vi "makeDecisions.vi"(8 "error in (no error)":errorcluster, 10 "model":refnum<class "Model.lvclass">, 11 "WaitingForSettledPState in":refnum<class "WaitingForSettledPState.lvclass">) -> (0 "error out":errorcluster, 2 "model 2":refnum<class "Model.lvclass">, 3 "WaitingForSettledPState out":refnum<class "WaitingForSettledPState.lvclass">)   [LabVIEW 2015, in "WaitingForSettledPState.lvclass"]
uses:
  WaitingForSettledPState.lvclass
  Model/Model/Model.lvclass
  Typedefs/StateSelector.ctl
  PreconditioningState/PreconditioningState.lvclass
  Typedefs/M1M3SSSTypedefs.lvlib
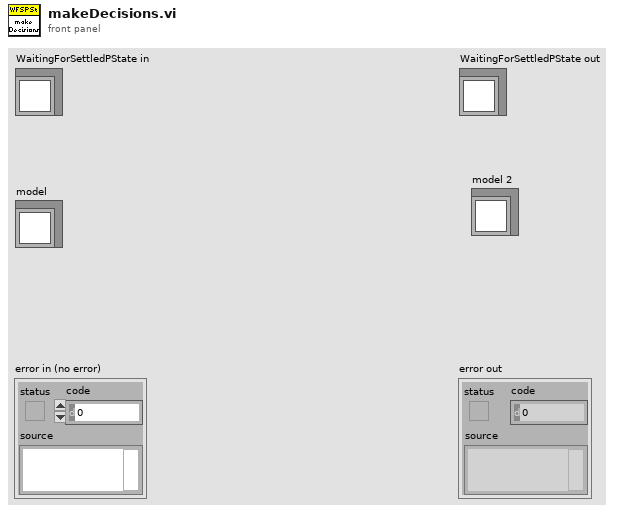
[diagram p1: front panel]
types:
  T1 = typedef "M1M3SSSTypedefs.lvlib/StateSelector.ctl" = enum16{"FaultState", "OffState", "RampingUpPressurePState", "RampingUpPressureSTState", "StandbyState", "StoppedState", "WaitingForSettledPState", "WaitingForSettledSTState"}
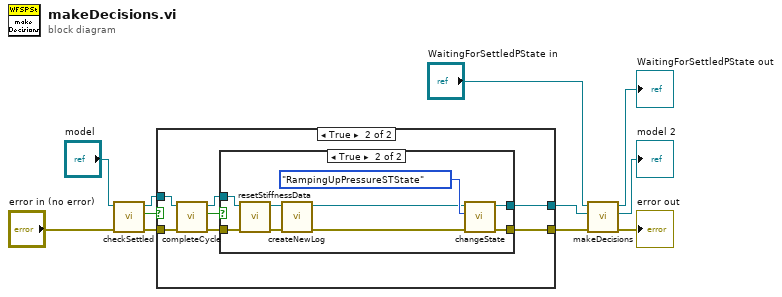
[diagram p0: block diagram]
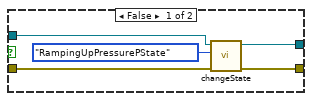
[diagram p3: hidden frame]
diagram:
  n1 = call "checkSettled.vi"("error in (no error)"="error in (no error)", "Model in"="model") -> ("error out"=w4:errorcluster, "settledIsTrue"=w1:bool, "Model out"=w2:refnum<class "Model.lvclass">)  [unwired: 7 in]
  n2 = case shown="True" w1 {
    tunnel: [w13 w19] -> w5
    tunnel: w4 -> [w13 w14]
    tunnel: [w12 w20] -> w3
    tunnel: w2 -> [w12 w15]
    frame False {
    }
    frame True {
      n3 = call "completeCycle.vi"("error in (no error)"=w14, "Model in"=w15) -> ("error out"=w16:errorcluster, "preconditiongCompleteIsTrue"=w18:bool, "Model out"=w17:refnum<class "Model.lvclass">)  [unwired: 7 in]
      n4 = case shown="True" w18 {
        tunnel: [w25 w34] -> w20
        tunnel: [w24 w33] -> w19
        tunnel: w17 -> [w22 w31]
        tunnel: w16 -> [w21 w30]
        frame False {
          n5 = call "changeState.vi"("error in (no error)"=w21, "State:"=StateSelector."RampingUpPressurePState", "Model in"=w22) -> ("error out"=w24:errorcluster, "Model out"=w25:refnum<class "Model.lvclass">)  [unwired: 7 in]
        }
        frame True {
          n6 = call "resetStiffnessData.vi"("error in (no error)"=w30, "Model in"=w31) -> ("error out"=w28:errorcluster, "Model out"=w29:refnum<class "Model.lvclass">)  [unwired: 8 in]
          n7 = call "createNewLog.vi"("error in (no error)"=w28, "Model in"=w29) -> ("error out"=w26:errorcluster, "Model out"=w27:refnum<class "Model.lvclass">)  [unwired: 8 in]
          n8 = call "changeState.vi"("error in (no error)"=w26, "State:"=StateSelector."RampingUpPressureSTState", "Model in"=w27) -> ("error out"=w33:errorcluster, "Model out"=w34:refnum<class "Model.lvclass">)  [unwired: 7 in]
        }
      }
    }
  }
  n9 = call-parent "makeDecisions.vi"("error in (no error)"=w5, "model"=w3, "EnabledState in"="WaitingForSettledPState in") -> ("error out"=→"error out":errorcluster, "model 2"=→"model 2":refnum<class "Model.lvclass">, "EnabledState out"=→"WaitingForSettledPState out":refnum<class "WaitingForSettledPState.lvclass">)  [unwired: 6 in]
